vi "VisionControl.vi"() -> ()   [LabVIEW 2015]
uses:
  <vilib>/vision/driver/IMAQdx.llb/IMAQdx Camera Control Mode.ctl
  SupportCode/GlobalVars.vi
  <vilib>/vision/driver/NI_Vision_Acquisition_Software.lvlib
panel:
  in  "AllowedDeviation":dbl=0.37 format="%#_13g"
  out "TargetDistance":dbl
  in  "HorizontalOffset":dbl=18.0
  out "Image":T1(plugin-control)
  out "Gyro Setpoint Vs. Actual":dynamicdata(graph)
  out "DesiredGyroValue":dbl
  out "CurrentGyroValue":dbl
  out "TargetRight":bool
  out "TargetLeft":bool
  out "OnTarget":bool
  out "VisionLoopRate":dbl
  out "Particle Measurements (Pixels) (Particle Analysis 1)":dbl[][](array[numeric]) format="%.2f"
  out "Number of Particles (Particle Analysis 1)":i32
  in  "Save":bool
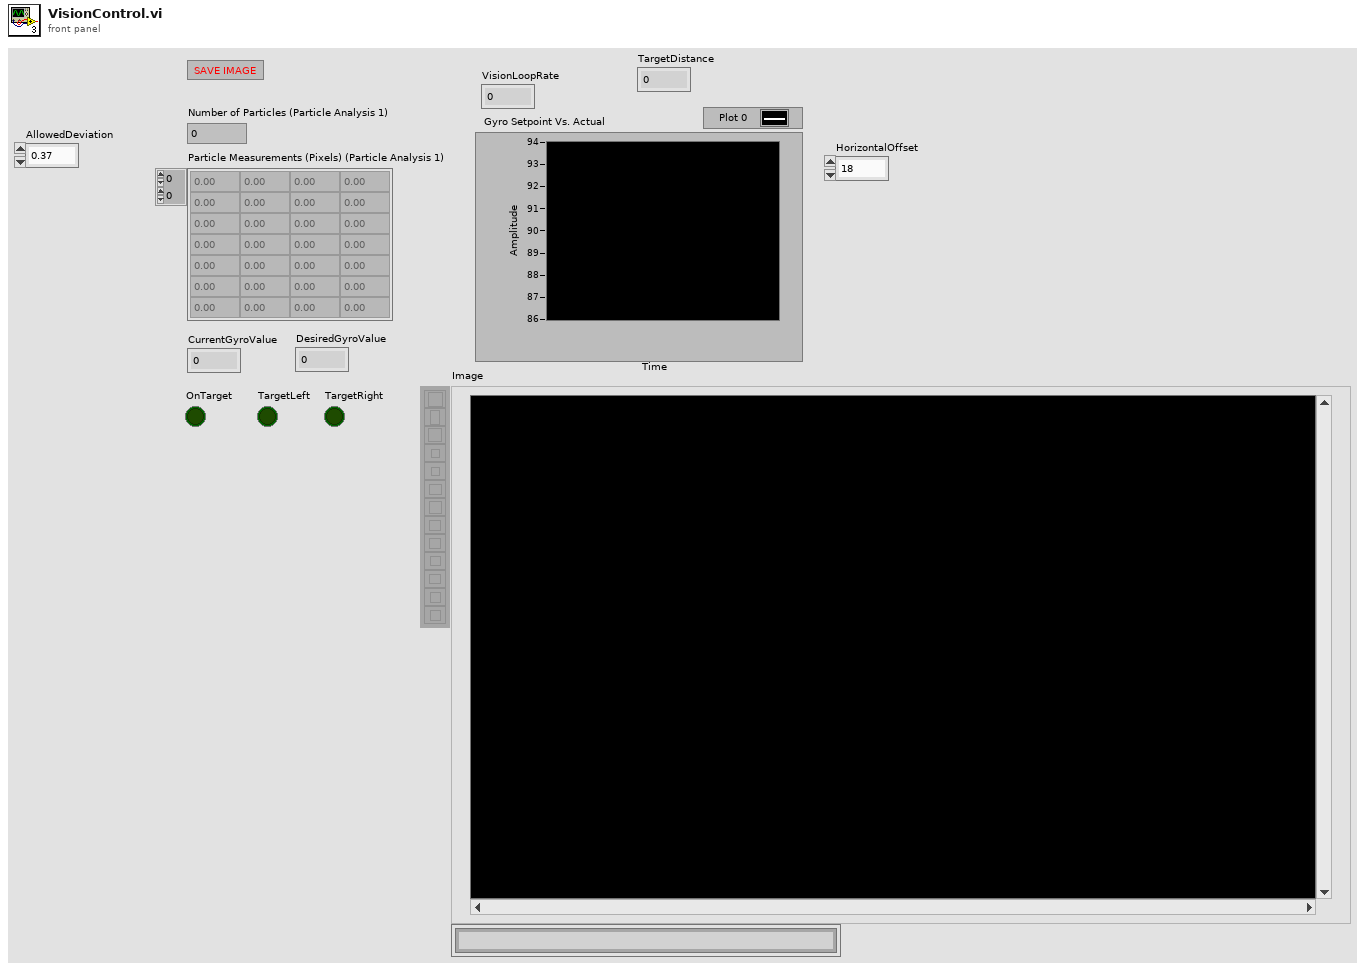
[diagram p1: front panel]
types:
  T1 = typedef "IMAQ Image.ctl" = refnum<image>
  T2 = typedef "Image Type" = u32
  T3 = typedef "NI_Vision_Acquisition_Software.lvlib/IMAQdx Camera Control Mode.ctl" = enum32{"Controller", "Listener"}
  T4 = cluster{"Type":u32, "Version":u32, "Flags":u32, "SerialNumberHigh":u32, "SerialNumberLow":u32, "BusType":u32, "InterfaceName":string, "VendorName":string, "ModelName":string, "CameraFileName":string, "CameraAttributeURL":string}[]
  T5 = cluster{"Type":u32, "Version":u32, "Flags":u32, "SerialNumberHigh":u32, "SerialNumberLow":u32, "BusType":u32, "InterfaceName":string, "VendorName":string, "ModelName":string, "CameraFileName":string, "CameraAttributeURL":string}
  T6 = typedef "IMAQdx.ctl" = refnum<k21>
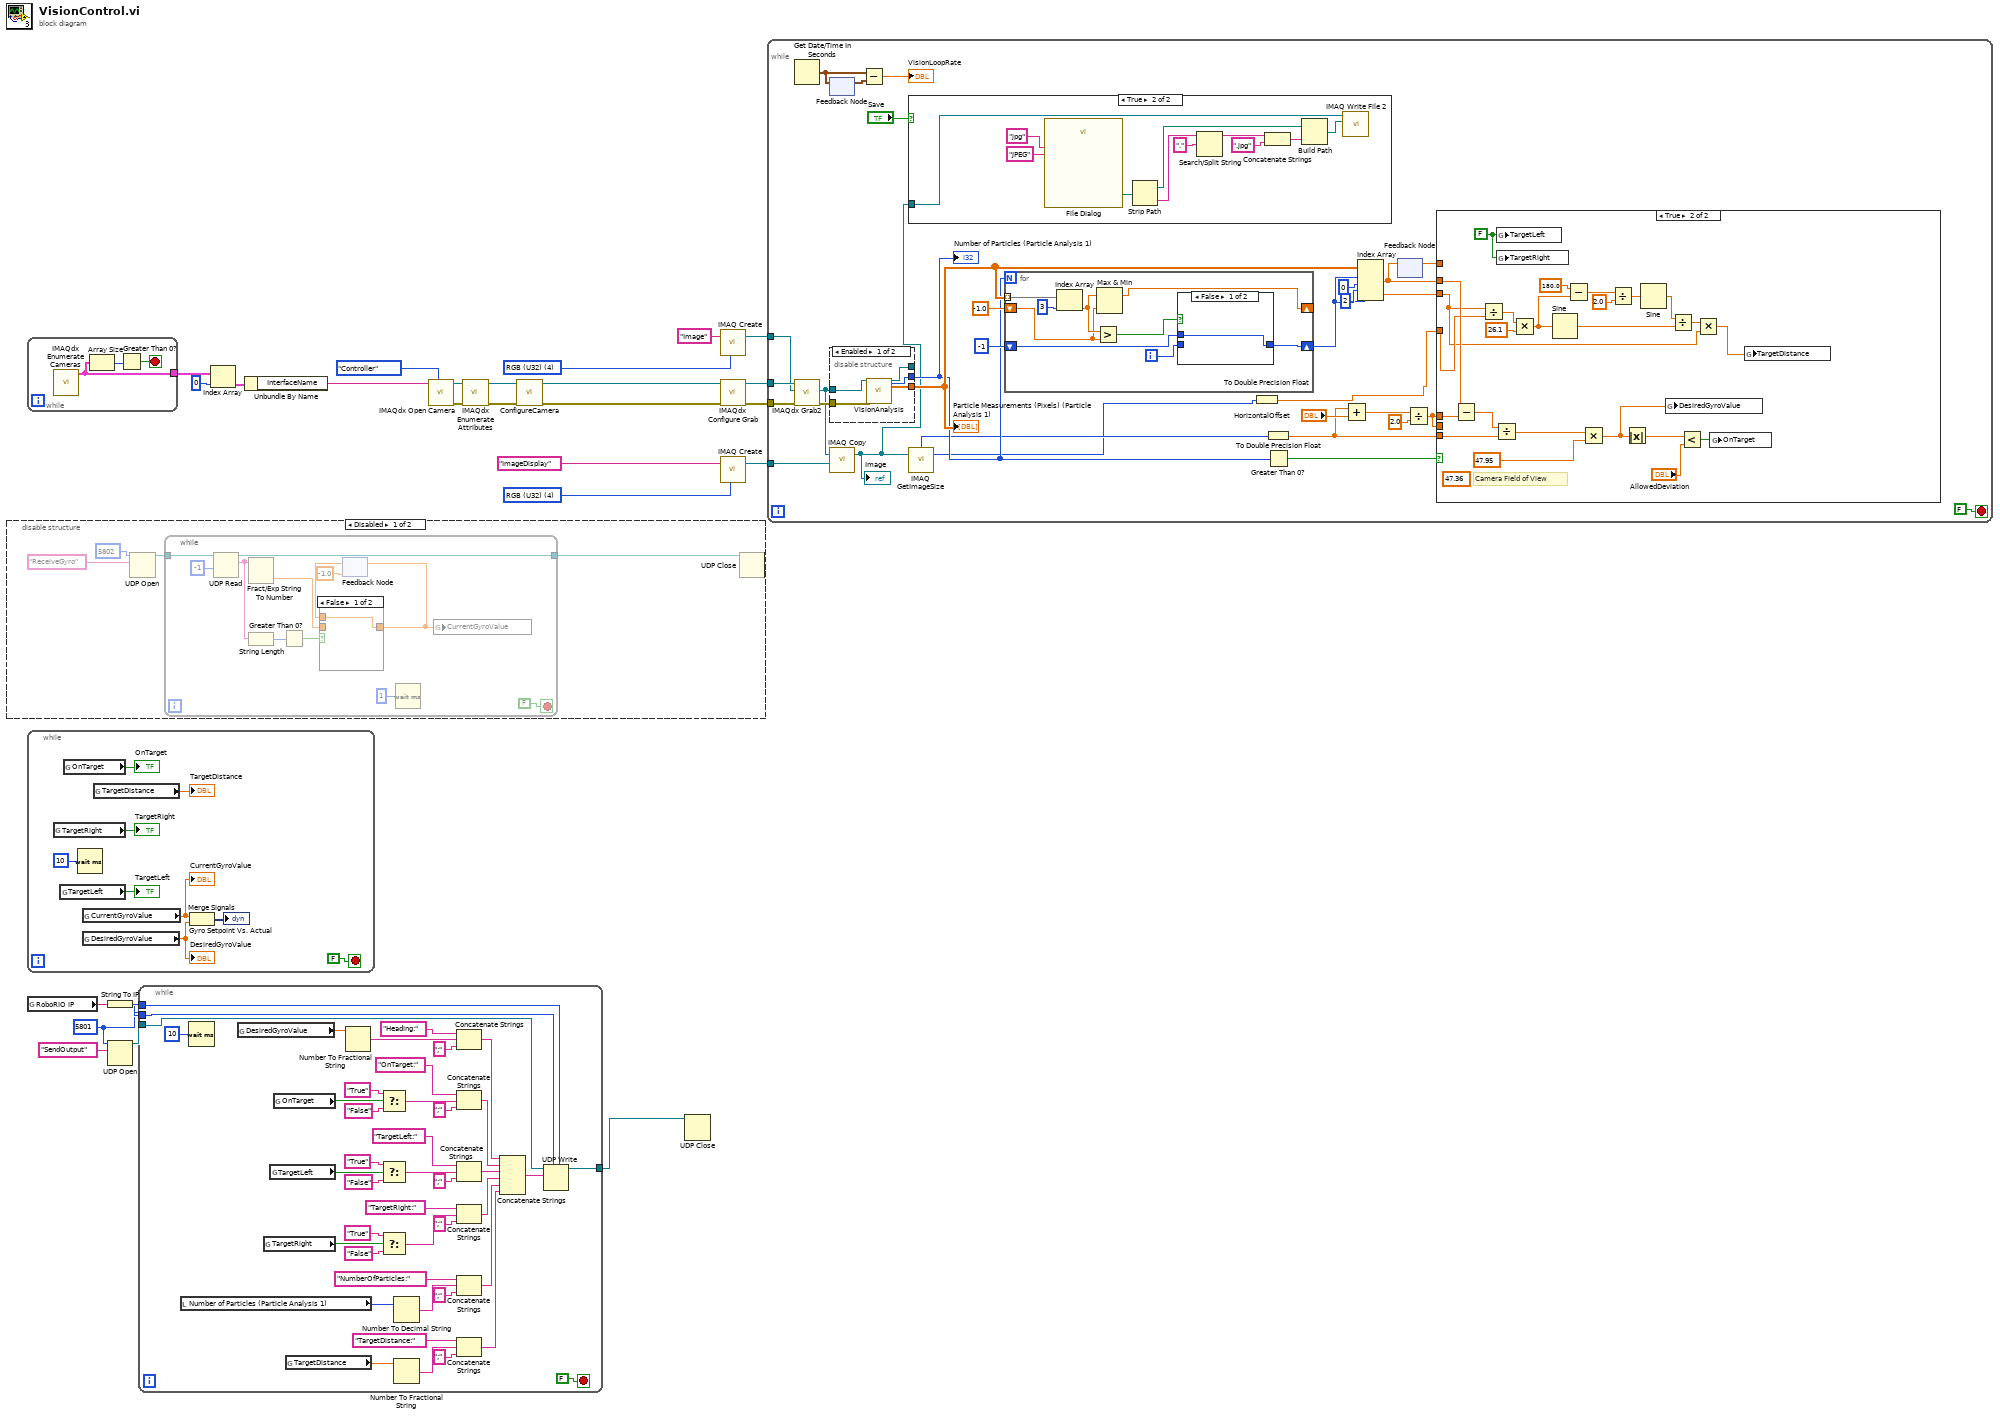
[diagram p0: block diagram]
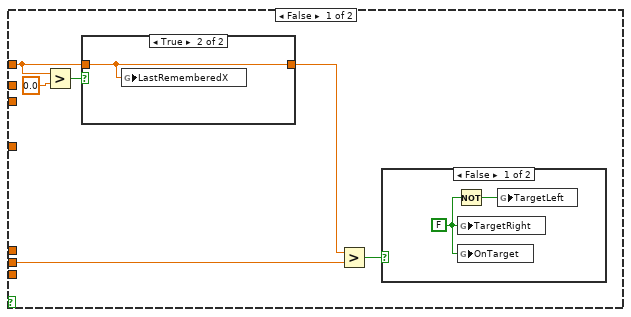
[diagram p5: hidden frame]
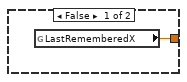
[diagram p6: hidden frame]
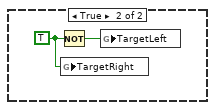
[diagram p7: hidden frame]
diagram:
  w2 = T2 4 items=["Grayscale (U8)", "Grayscale (I16)", "Grayscale (SGL)", "Complex (CSG)", "RGB (U32)", "HSL (U32)", "RGB (U64)", "Grayscale (U16)"] ("Image Type")
  w12 = T2 4 items=["Grayscale (U8)", "Grayscale (I16)", "Grayscale (SGL)", "Complex (CSG)", "RGB (U32)", "HSL (U32)", "RGB (U64)", "Grayscale (U16)"] ("Image Type")
  w21 = u16 5801 ("port")
  n1 = disable-structure shown="Disabled" {
    frame Disabled {
      n2 = UDP Open(10:"ReceiveGyro" ("service name"), 11:u16 5802 ("port")) -> (port=w27:refnum<k16>)  [unwired: 3 in, 2 out]
      n3 = while {
        tunnel: w27 -> [w41]
        tunnel: [w40] -> w26
        stop <- FALSE stop-if-true
        n4 = UDP Read(connection ID=w41, timeout ms (25000)=-1) -> (data out=w35:string, 3:w40:refnum<k16>)  [unwired: 2 in, 3 out]
        n5 = Fract/Exp String To Number(string=w35) -> (number=w34:dbl)  [unwired: 3 in, 1 out]
        n6 = String Length(string=w35) -> (length=w37:i32)
        n7 = Greater Than 0?(x=w37) -> (x > 0?=w36:bool)
        n8 = feedback #1(-1.0) -> (w32:dbl)
        n9 = case shown="False" w36 {
          tunnel: w34 -> [_ w43]
          tunnel: [w42 w43] -> w33
          tunnel: w32 -> [w42 _]
          frame False {
          }
          frame True {
          }
        }
        n10 = feedback-in #1(w33) -> ()
        n11 = Wait (ms)(milliseconds to wait=u32 1) -> ()  [unwired: 1 out]
        n12 = global write "GlobalVars.vi" "CurrentGyroValue"(w33) -> ()
      }
      n13 = UDP Close(connection ID=w26) -> ()  [unwired: 1 in, 2 out]
    }
    frame Enabled {
    }
  }
  n14 = while {
    tunnel: [w44] -> w19
    stop <- w45 stop-if-true
    n15 = call <vilib>:"IMAQdx Enumerate Cameras.vi"() -> ("Camera Information Array"=w44:T4)  [unwired: 10 in, 1 out]
    n16 = Array Size(array=w44) -> (size(s)=w46:i32)
    n17 = Greater Than 0?(x=w46) -> (x > 0?=w45:bool)
  }
  n18 = while {
    stop <- FALSE stop-if-true
    n19 = global read "GlobalVars.vi" "TargetRight"() -> (→"TargetRight":bool)
    n20 = global read "GlobalVars.vi" "TargetLeft"() -> (→"TargetLeft":bool)
    n21 = global read "GlobalVars.vi" "OnTarget"() -> (→"OnTarget":bool)
    n22 = Wait (ms)(milliseconds to wait=u32 10) -> ()  [unwired: 1 out]
    n23 = global read "GlobalVars.vi" "CurrentGyroValue"() -> (w49:dbl)
    "CurrentGyroValue" <- w49
    n24 = global read "GlobalVars.vi" "DesiredGyroValue"() -> (w48:dbl)
    "DesiredGyroValue" <- w48
    n25 = global read "GlobalVars.vi" "TargetDistance"() -> (→"TargetDistance":dbl)
    n26 = Merge Signals(w49, w48) -> (→"Gyro Setpoint Vs. Actual":dynamicdata)
  }
  n27 = global read "GlobalVars.vi" "RoboRIO IP"() -> (w23:string)
  n28 = String To IP(1:w23) -> (0:w22:u32)
  n29 = UDP Open(10:"SendOutput" ("service name"), 11:w21) -> (port=w24:refnum<k16>)  [unwired: 3 in, 2 out]
  n30 = while {
    tunnel: w24 -> [w66]
    tunnel: w22 -> [w77]
    tunnel: w21 -> [w76]
    tunnel: [w78] -> w20
    stop <- FALSE stop-if-true
    n31 = local read "Number of Particles (Particle Analysis 1)"() -> (w63:i32)
    n32 = Wait (ms)(milliseconds to wait=u32 10) -> ()  [unwired: 1 out]
    n33 = global read "GlobalVars.vi" "DesiredGyroValue"() -> (w96:dbl)
    n34 = global read "GlobalVars.vi" "TargetRight"() -> (w82:bool)
    n35 = global read "GlobalVars.vi" "TargetLeft"() -> (w87:bool)
    n36 = global read "GlobalVars.vi" "OnTarget"() -> (w92:bool)
    n37 = global read "GlobalVars.vi" "TargetDistance"() -> (w56:dbl)
    n38 = Number To Fractional String(number=w96) -> (F-format string=w95:string)  [unwired: 3 in]
    n39 = Select(t="True" ("string"), s=w92, f="False") -> (s? t:f=w91:string)
    n40 = Select(t="True" ("string"), s=w87, f="False") -> (s? t:f=w86:string)
    n41 = Select(t="True" ("string"), s=w82, f="False") -> (s? t:f=w81:string)
    n42 = Number To Decimal String(number=w63) -> (decimal integer string=w62:string)  [unwired: 1 in]
    n43 = Number To Fractional String(number=w56) -> (F-format string=w57:string)  [unwired: 3 in]
    n44 = Concatenate Strings("Heading:" ("string"), w95, ";" ("string")) -> (w71:string)
    n45 = Concatenate Strings("OnTarget:" ("string"), w91, ";" ("string")) -> (w70:string)
    n46 = Concatenate Strings("TargetLeft:" ("string"), w86, ";" ("string")) -> (w69:string)
    n47 = Concatenate Strings("TargetRight:" ("string"), w81, ";" ("string")) -> (w68:string)
    n48 = Concatenate Strings("NumberOfParticles:" ("string"), w62, ";" ("string")) -> (w61:string)
    n49 = Concatenate Strings("TargetDistance:" ("string"), w57, ";" ("string")) -> (w58:string)
    n50 = Concatenate Strings(w71, w70, w69, w68, w61, w58) -> (w67:string)
    n51 = UDP Write(address=w77, port or service name=w76, connection ID=w66, data in=w67) -> (3:w78:refnum<k16>)  [unwired: 2 in, 1 out]
  }
  n52 = Index Array(array=w19, index=0) -> (element=w17:T5)
  n53 = Unbundle By Name(w17) -> ("InterfaceName"=w16:string)
  n54 = call <vilib>:"IMAQdx Open Camera.vi"("Camera Control Mode"=IMAQdx_Camera_Control_Mode."Controller", "Session In"=w16) -> ("error out"=w11:errorcluster, "Session Out"=w10:T6)  [unwired: 8 in]
  n55 = call <vilib>:"IMAQdx Enumerate Attributes.vi"("error in"=w11, "Session In"=w10) -> ("error out"=w8:errorcluster, "Session Out"=w9:T6)  [unwired: 7 in, 1 out]
  n56 = call "ConfigureCamera.vi"("error in (no error)"=w8, "Refnum in"=w9) -> ("error out"=w5:errorcluster, "Refnum out"=w6:T6)  [unwired: 8 in]
  n57 = UDP Close(connection ID=w20) -> ()  [unwired: 1 in, 2 out]
  n58 = call "IMAQ Create"("Image Name"="Image", "Image Type"=w12) -> ("New Image"=w14:T1)  [unwired: 3 in, 1 out]
  n59 = call <vilib>:"IMAQdx Configure Grab.vi"("error in"=w5, "Session In"=w6) -> ("error out"=w4:errorcluster, "Session Out"=w7:T6)  [unwired: 8 in]
  n60 = call "IMAQ Create"("Image Name"="ImageDisplay", "Image Type"=w2) -> ("New Image"=w1:T1)  [unwired: 3 in, 1 out]
  n61 = while {
    tunnel: w14 -> [w117]
    tunnel: w7 -> [w118]
    tunnel: w4 -> [w116]
    tunnel: w1 -> [w112]
    stop <- FALSE stop-if-true
    n62 = Get Date/Time In Seconds() -> (seconds since 1Jan1904=w121:timestamp)
    n63 = call <vilib>:"IMAQdx Grab2.vi"("error in"=w116, "Image In"=w117, "Session In"=w118) -> ("error out"=w115:errorcluster, "Image Out"=w111:T1)  [unwired: 5 in, 2 out]
    n64 = feedback-in #2(w121) -> ()
    n65 = feedback #2() -> (w120:timestamp)  [unwired: 1 in]
    n66 = disable-structure shown="Enabled" {
      disable-tunnel: w115 -> [w134 _]
      disable-tunnel: w111 -> [w133 _]
      disable-tunnel: [w132 _] -> w125
      disable-tunnel: [w131 _] -> w123
      disable-tunnel: [w130 _] -> _
      frame Enabled {
        n67 = call "VisionAnalysis.vi"("Image In"=w133, "error in"=w134) -> ("Image Out"=w130:T1, "Number of Particles (Particle Analysis 1)"=w131:i32, "Particle Measurements (Pixels) (Particle Analysis 1)"=w132:dbl[][])  [unwired: 22 in, 1 out]
      }
      frame Disabled {
      }
    }
    "Number of Particles (Particle Analysis 1)" <- w123
    "Particle Measurements (Pixels) (Particle Analysis 1)" <- w125
    n68 = call "IMAQ Copy"("Image Dst"=w112, "Image Src"=w111) -> ("Image Dst Out"=w110:T1)  [unwired: 4 in, 1 out]
    "Image" <- w110
    n69 = Subtract(x=w121, y=w120) -> (x-y=→"VisionLoopRate":dbl)
    n70 = case shown="True" "Save" {
      tunnel: w110 -> [_ w182]
      frame False {
      }
      frame True {
        n71 = call "File Dialog"("pattern (all files)"="jpg", "pattern label"="JPEG") -> ("selected path"=w190:path)  [unwired: 10 in, 3 out]
        n72 = Strip Path(path=w190) -> (stripped path=w189:path, name=w188:string)
        n73 = Search/Split String(string=w188, search string/char (-)=".") -> (substring before match=w186:string)  [unwired: 1 in, 2 out]
        n74 = Concatenate Strings(w186, ".jpg" ("string")) -> (w184:string)
        n75 = Build Path(base path=w189, name or relative path=w184) -> (appended path=w183:path)
        n76 = call-poly "IMAQ Write File 2"("File Path"=w183, "Image"=w182) -> ()  [unwired: 8 in, 2 out]
      }
    }
    n77 = call "IMAQ GetImageSize"("Image"=w110) -> ("Y Resolution"=w101:i32, "X Resolution"=w109:i32)  [unwired: 3 in, 1 out]
    n78 = for {
      N: w123 -> [_]
      tunnel: w125 -> [w179] mode=indexing
      shift-right: [w177] -> _
      shift-left: -1.0 -> [w175]
      shift-right: [w172] -> w103
      shift-left: -1 -> [w171]
      i -> [w173]
      n79 = Index Array(array=w179, index=3) -> (element=w176:dbl)
      n80 = Greater?(x=w176, y=w175) -> (0:w174:bool)
      n81 = Max & Min(x=w176, y=w175) -> (max(x,y)=w177:dbl)  [unwired: 1 out]
      n82 = case shown="False" w174 {
        tunnel: w173 -> [_ w181]
        tunnel: [w180 w181] -> w172
        tunnel: w171 -> [w180 _]
        frame False {
        }
        frame True {
        }
      }
    }
    n83 = To Double Precision Float(number=w101) -> (double precision float=w100:dbl)
    n84 = To Double Precision Float(number=w109) -> (double precision float=w105:dbl)
    n85 = Greater Than 0?(x=w123) -> (x > 0?=w122:bool)
    n86 = Add(x=w105, y="HorizontalOffset") -> (x+y=w107:dbl)
    n87 = Index Array(array=w125, index (row) #1=w103, index (col) #1=0 ("disabled index (col)"), index (row) #2=w103, index (col) #2=2 ("disabled index (col)")) -> (element #1=w114:dbl, element #2=w99:dbl)
    n88 = feedback-in #3(w114) -> ()
    n89 = feedback #3() -> (w113:dbl)  [unwired: 1 in]
    n90 = Divide(x=w107, y=2.0) -> (x/y=w104:dbl)
    n91 = case shown="True" w122 {
      tunnel: w114 -> [_ w170]
      tunnel: w113 -> [w136 _]
      tunnel: w104 -> [w135 _]
      tunnel: w105 -> [_ w162]
      tunnel: w104 -> [_ w161]
      tunnel: w100 -> [_ w159]
      tunnel: w99 -> [_ w149]
      frame False {
        n92 = Greater?(x=w136, y=0.0) -> (0:w138:bool)
        n93 = case shown="True" w138 {
          tunnel: w136 -> [_ w142]
          tunnel: [w141 w142] -> w137
          frame False {
            n94 = global read "GlobalVars.vi" "LastRememberedX"() -> (w141:dbl)
          }
          frame True {
            n95 = global write "GlobalVars.vi" "LastRememberedX"(w142) -> ()
          }
        }
        n96 = Greater?(x=w137, y=w135) -> (0:w140:bool)
        n97 = case shown="False" w140 {
          frame False {
            w143 = FALSE ("TargetRight")
            n98 = Not(x=w143) -> (.not. x?=w144:bool)
            n99 = global write "GlobalVars.vi" "TargetRight"(w143) -> ()
            n100 = global write "GlobalVars.vi" "OnTarget"(w143) -> ()
            n101 = global write "GlobalVars.vi" "TargetLeft"(w144) -> ()
          }
          frame True {
            w146 = TRUE ("TargetRight")
            n102 = Not(x=w146) -> (.not. x?=w145:bool)
            n103 = global write "GlobalVars.vi" "TargetRight"(w146) -> ()
            n104 = global write "GlobalVars.vi" "TargetLeft"(w145) -> ()
          }
        }
      }
      frame True {
        (unwired) 47.36 ("y")
        w163 = FALSE ("TargetRight")
        # "Camera Field of View"
        n105 = Subtract(x=w170, y=w161) -> (x-y=w169:dbl)
        n106 = Divide(x=w149, y=w159) -> (x/y=w158:dbl)
        n107 = Divide(x=w169, y=w162) -> (x/y=w168:dbl)
        n108 = global write "GlobalVars.vi" "TargetLeft"(w163) -> ()
        n109 = global write "GlobalVars.vi" "TargetRight"(w163) -> ()
        n110 = Multiply(x=w158, y=26.1) -> (x*y=w153:dbl)
        n111 = Sine(x=w153) -> (sin(x)=w151:dbl)
        n112 = Subtract(x=180.0, y=w153) -> (x-y=w156:dbl)
        n113 = Multiply(x=w168, y=47.95) -> (x*y=w147:dbl)
        n114 = Divide(x=w156, y=2.0) -> (x/y=w154:dbl)
        n115 = Absolute Value(x=w147) -> (abs(x)=w164:dbl)
        n116 = Sine(x=w154) -> (sin(x)=w152:dbl)
        n117 = global write "GlobalVars.vi" "DesiredGyroValue"(w147) -> ()
        n118 = Divide(x=w152, y=w151) -> (x/y=w150:dbl)
        n119 = Less?(x=w164, y="AllowedDeviation") -> (x < y?=w165:bool)
        n120 = Multiply(x=w150, y=w149) -> (x*y=w148:dbl)
        n121 = global write "GlobalVars.vi" "OnTarget"(w165) -> ()
        n122 = global write "GlobalVars.vi" "TargetDistance"(w148) -> ()
      }
    }
  }
